vi "Post Handle.vi"(8 "Error in":errorcluster, 9 "Was Msg":bool, 10 "Has Handled":bool, 11 "TEMPLATE Actor in":refnum<class "TEMPLATE Actor.lvclass">) -> (0 "Error out":errorcluster, 3 "TEMPLATE Actor out":refnum<class "TEMPLATE Actor.lvclass">)   [LabVIEW 2020, in "_Template.lvlib" / "Templates.lvlib" / "TEMPLATE Actor.lvlib" / "TEMPLATE Actor.lvclass"]
uses:
  TEMPLATE Actor.lvclass
  TEMPLATE Actor.lvclass/TEMPLATE Actor.ctl
  jettl/jettl/Actor/Actor/Actor.lvclass
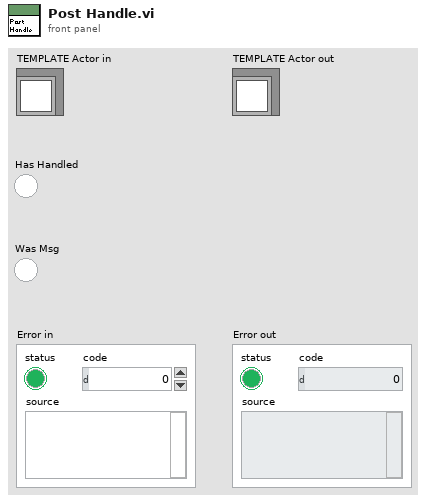
[diagram p1: front panel]
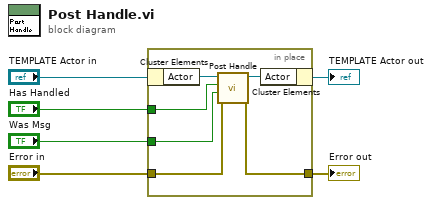
[diagram p0: block diagram]
diagram:
  n1 = in-place {
    in-place-border: "Error in" -> [w10]
    in-place-border: [w9] -> w3
    in-place-border: "Has Handled" -> [w8]
    in-place-border: "Was Msg" -> [w7]
    n2 = in-place-cluster #1("TEMPLATE Actor in") -> ("Actor"=w12:refnum<class "Actor.lvclass">)
    n3 = call-dynamic "Post Handle.vi"("Error in"=w10, "Was Msg"=w7, "Has Handled"=w8, "Actor in"=w12) -> ("Error out"=w9:errorcluster, "Actor out"=w11:refnum<class "Actor.lvclass">)  [unwired: 6 in]
    n4 = in-place-cluster #1("Actor"=w11) -> (→"TEMPLATE Actor out":refnum<class "TEMPLATE Actor.lvclass">)
  }
  "Error out" <- w3
